vi "arduino-json-messenger.vi"() -> ()   [LabVIEW 2024]
uses:
  <vilib>/Instr/_visa.llb/VISA Configure Serial Port (Instr).vi
panel:
  in  "stop":bool
  in  "Start/Update":bool
  in  "Manual Command Entry":string
  in  "Print Option":string(combo)="all"
  in  "Speed/Offset":i16
  in  "Column":string(combo)="0"
  in  "Row":string(combo)="A"
  in  "Command":T1(ring)
  in  "baud rate 115200":u32=115200
  in  "VISA resource name":refnum<visa-resource-name>="COM29"
  out "Num Bytes Rx":u32
  out "error out":errorcluster
  out "json-cmd":string
  in  "send-cmd":bool
  out "Arduino - Output":string
  in  "exit":bool
  # "ALI-J"
  # "Arduino Labview Interface - JSON"
  # "Data"
  # "{\"cmd\":\"Set offset for fan (at current speed)  -> \"}\n   {\"A0\": -4096 to 4095}\n   {\"C3\": -4096 to 4095}\n\n{\"cmd\":\"Set Global Fan Speed  -> \"}\n   {\"speed\": 0 to 4095}\n\n{\"cmd\":\"Start & Stop Fans  -> \"}\n   {\"start\":0}\n   {\"stop\":0}\n\n{\"cmd\":\"Set Operational Modes ->\"}\n   {\"cal\":\"\"}\n   {\"run\":\"\"}\n\n{\"cmd\":\"View/Save/Delete Data ->\"}\n   {\"save\":\"\"}\n   {\"del\":0 to 4095}\n   {\"print\":\"all\"}\n   {\"print\":\"pwm\"}\n   {\"get\":0 to 4095}\n   {\"help\":\"\"}"
  # "Command Builder"
  # "Serial Options"
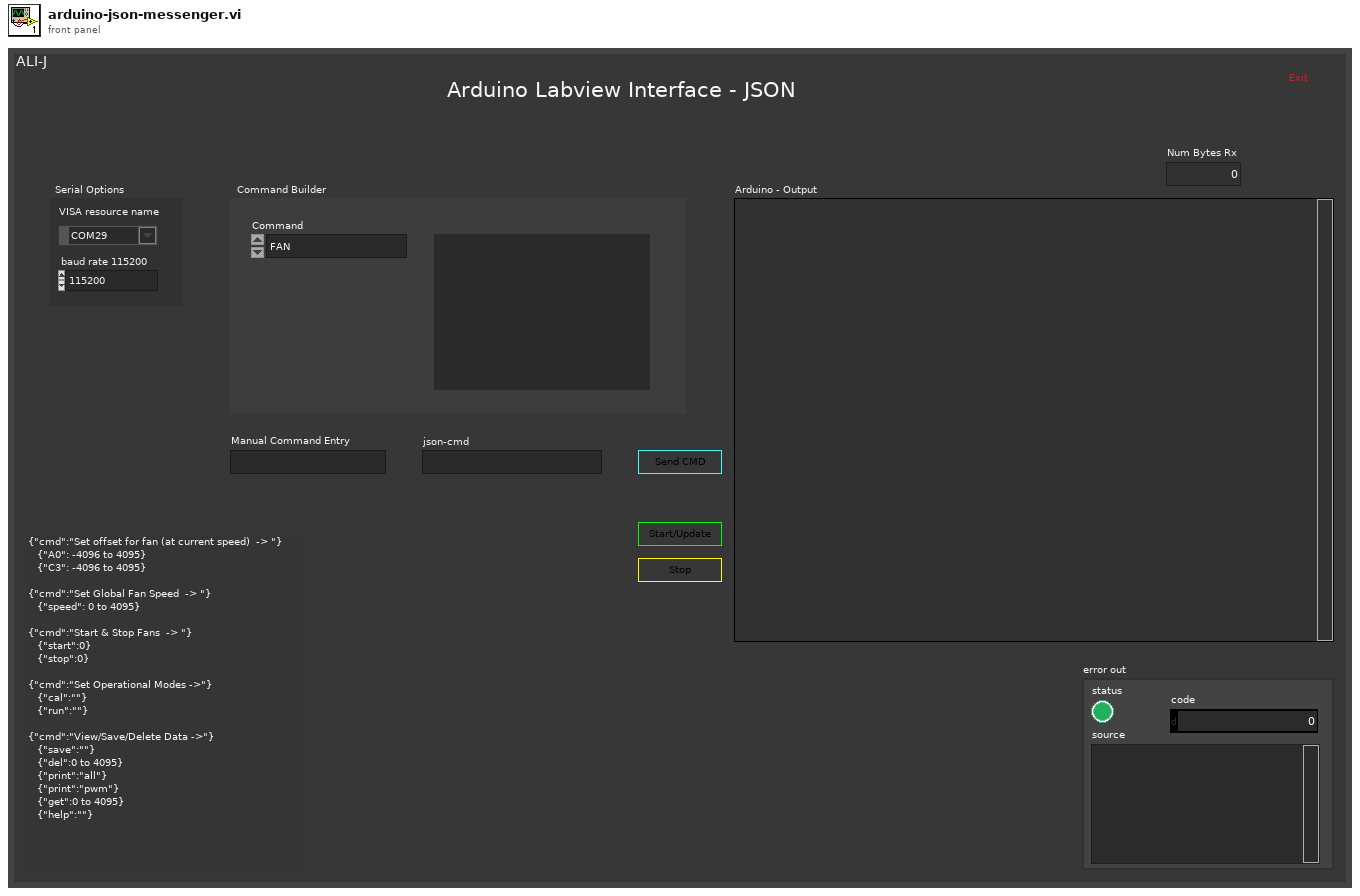
[diagram p1: front panel]
types:
  T1 = enum16{"FAN", "SPEED", "START", "STOP", "CALIBRATE", "RUN", "SAVE", "DELETE", "PRINT", "GET", "HELP", "none"}
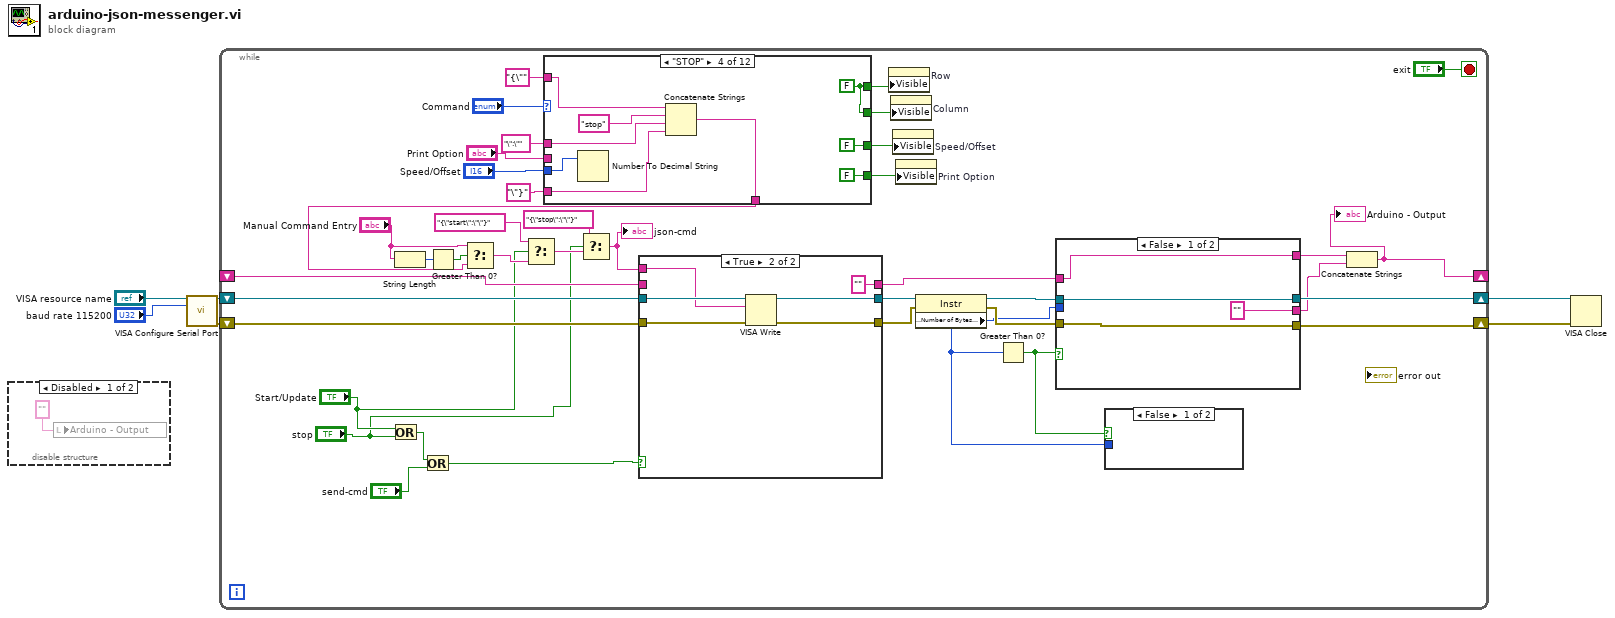
[diagram p0: block diagram]
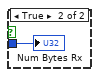
[diagram p3: hidden frame]
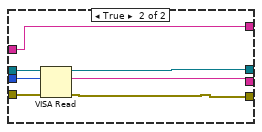
[diagram p4: hidden frame]
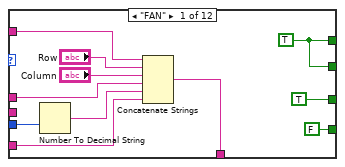
[diagram p6: hidden frame]
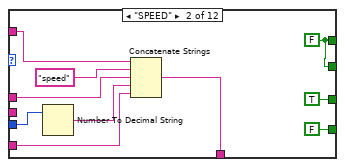
[diagram p7: hidden frame]
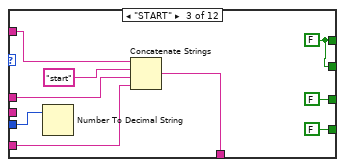
[diagram p8: hidden frame]
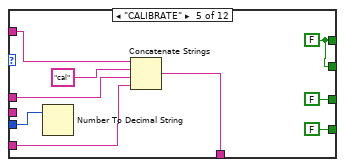
[diagram p9: hidden frame]
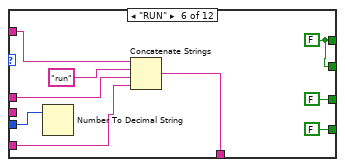
[diagram p10: hidden frame]
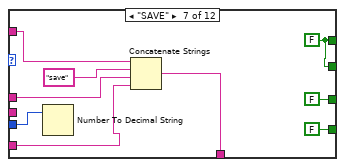
[diagram p11: hidden frame]
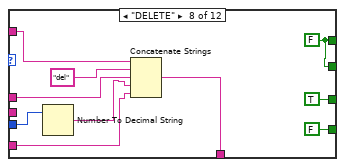
[diagram p12: hidden frame]
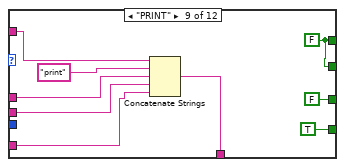
[diagram p13: hidden frame]
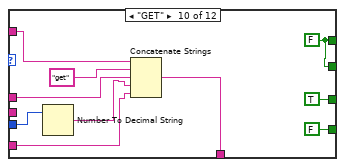
[diagram p14: hidden frame]
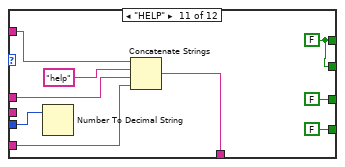
[diagram p15: hidden frame]
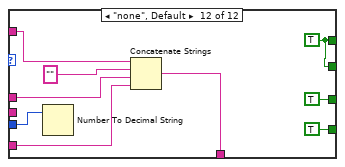
[diagram p16: hidden frame]
diagram:
  n1 = disable-structure shown="Disabled" {
    frame Disabled {
      n2 = local write "Arduino - Output"("" ("string")) -> ()
    }
    frame Enabled {
    }
  }
  n3 = call-poly "VISA Configure Serial Port"("VISA resource name"="VISA resource name", "baud rate (9600)"="baud rate 115200") -> ("VISA resource name out"=w5:refnum<visa-resource-name>, "error out"=w4:errorcluster)  [unwired: 12 in]
  n4 = while {
    shift-right: [w45] -> w3
    shift-left: w5 -> [w37]
    shift-right: [w24] -> w1
    shift-left: w4 -> [w35]
    shift-right: [w25] -> _
    shift-left: _ -> [w26]
    stop <- "exit" stop-if-true
    n5 = Or(x="Start/Update", y="stop") -> (x .or. y?=w16:bool)
    n6 = String Length(string="Manual Command Entry") -> (length=w21:i32)
    n7 = Or(x=w16, y="send-cmd") -> (x .or. y?=w17:bool)
    n8 = Greater Than 0?(x=w21) -> (x > 0?=w20:bool)
    n9 = case shown="\"STOP\"" "Command" {
      tunnel: [w79 w89 w98 w107 w116 w125 w134 w144 w153 w163 w172 w181] -> w42
      tunnel: [w79 w89 w98 w107 w116 w125 w134 w144 w153 w163 w172 w181] -> w41
      tunnel: "Speed/Offset" -> [w75 w85 w94 w103 w112 w121 w130 w140 _ w159 w168 w177]
      tunnel: "{\"" -> [w74 w88 w97 w106 w115 w124 w133 w143 w152 w162 w171 w180]
      tunnel: "\":\"" -> [w73 w86 w95 w104 w113 w122 w131 w141 w150 w160 w169 w178]
      tunnel: [w72 w82 w93 w102 w111 w120 w129 w139 w149 w158 w167 w176] -> w18
      tunnel: "\"}" -> [w71 w83 w92 w101 w110 w119 w128 w136 w147 w155 w165 w175]
      tunnel: [TRUE ("Visible") TRUE ("Visible") FALSE ("Visible") FALSE ("Visible") FALSE ("Visible") FALSE ("Visible") FALSE ("Visible") TRUE ("Visible") FALSE ("Visible") TRUE ("Visible") FALSE ("Visible") TRUE ("Visible")] -> w32
      tunnel: [FALSE ("Visible") FALSE ("Visible") FALSE ("Visible") FALSE ("Visible") FALSE ("Visible") FALSE ("Visible") FALSE ("Visible") FALSE ("Visible") TRUE ("Visible") FALSE ("Visible") FALSE ("Visible") TRUE ("Visible")] -> w23
      tunnel: "Print Option" -> [_ _ _ _ _ _ _ _ w145 _ _ _]
      frame "FAN" {
        w79 = TRUE ("Visible")
        n10 = Number To Decimal String(number=w75) -> (decimal integer string=w76:string)  [unwired: 1 in]
        n11 = Concatenate Strings(w74, "Row", "Column", w73, w76, w71) -> (w72:string)
      }
      frame "SPEED" {
        w89 = FALSE ("Visible")
        n12 = Number To Decimal String(number=w85) -> (decimal integer string=w84:string)  [unwired: 1 in]
        n13 = Concatenate Strings(w88, "speed" ("string"), w86, w84, w83) -> (w82:string)
      }
      frame "START" {
        w98 = FALSE ("Visible")
        n14 = Number To Decimal String(number=w94) -> ()  [unwired: 1 in, 1 out]
        n15 = Concatenate Strings(w97, "start" ("string"), w95, w92) -> (w93:string)
      }
      frame "STOP" {
        w107 = FALSE ("Visible")
        n16 = Number To Decimal String(number=w103) -> ()  [unwired: 1 in, 1 out]
        n17 = Concatenate Strings(w106, "stop" ("string"), w104, w101) -> (w102:string)
      }
      frame "CALIBRATE" {
        w116 = FALSE ("Visible")
        n18 = Number To Decimal String(number=w112) -> ()  [unwired: 1 in, 1 out]
        n19 = Concatenate Strings(w115, "cal" ("string"), w113, w110) -> (w111:string)
      }
      frame "RUN" {
        w125 = FALSE ("Visible")
        n20 = Number To Decimal String(number=w121) -> ()  [unwired: 1 in, 1 out]
        n21 = Concatenate Strings(w124, "run" ("string"), w122, w119) -> (w120:string)
      }
      frame "SAVE" {
        w134 = FALSE ("Visible")
        n22 = Number To Decimal String(number=w130) -> ()  [unwired: 1 in, 1 out]
        n23 = Concatenate Strings(w133, "save" ("string"), w131, w128) -> (w129:string)
      }
      frame "DELETE" {
        w144 = FALSE ("Visible")
        n24 = Number To Decimal String(number=w140) -> (decimal integer string=w137:string)  [unwired: 1 in]
        n25 = Concatenate Strings(w143, "del" ("string"), w141, w137, w136) -> (w139:string)
      }
      frame "PRINT" {
        w153 = FALSE ("Visible")
        n26 = Concatenate Strings(w152, "print" ("string"), w150, w145, w147) -> (w149:string)
      }
      frame "GET" {
        w163 = FALSE ("Visible")
        n27 = Number To Decimal String(number=w159) -> (decimal integer string=w156:string)  [unwired: 1 in]
        n28 = Concatenate Strings(w162, "get" ("string"), w160, w156, w155) -> (w158:string)
      }
      frame "HELP" {
        w172 = FALSE ("Visible")
        n29 = Number To Decimal String(number=w168) -> ()  [unwired: 1 in, 1 out]
        n30 = Concatenate Strings(w171, "help" ("string"), w169, w165) -> (w167:string)
      }
      frame "none", Default {
        w181 = TRUE ("Visible")
        n31 = Number To Decimal String(number=w177) -> ()  [unwired: 1 in, 1 out]
        n32 = Concatenate Strings(w180, "" ("string"), w178, w175) -> (w176:string)
      }
    }
    n33 = Select(t="Manual Command Entry", s=w20, f=w18) -> (s? t:f=w14:string)
    n34 = Select(t="{\"start\":\"\"}", s="Start/Update", f=w14) -> (s? t:f=w13:string)
    n35 = Select(t="{\"stop\":\"\"}", s="stop", f=w13) -> (s? t:f=w12:string)
    "json-cmd" <- w12
    n36 = case shown="True" w17 {
      tunnel: w12 -> [_ w64]
      tunnel: w37 -> [w62 w68]
      tunnel: [w62 w67] -> w36
      tunnel: w35 -> [w61 w66]
      tunnel: [w61 w65] -> w34
      tunnel: [w60 ""] -> w27
      tunnel: w26 -> [w60 _]
      frame False {
      }
      frame True {
        n37 = VISA Write(VISA resource name=w68, write buffer=w64, error in (no error)=w66) -> (VISA resource name out=w67:refnum<visa-resource-name>, error out=w65:errorcluster)  [unwired: 1 out]
      }
    }
    n38 = property on="Row" class="CmbBox"("Visible"=w42) -> ()  [unwired: 2 in, 2 out]
    n39 = property on="Column" class="CmbBox"("Visible"=w41) -> ()  [unwired: 2 in, 2 out]
    n40 = property on="Speed/Offset" class="DigNum (strict)"("Visible"=w32) -> ()  [unwired: 2 in, 2 out]
    n41 = property on="Print Option" class="CmbBox"("Visible"=w23) -> ()  [unwired: 2 in, 2 out]
    n42 = property class="Instr"(reference=w36, error in=w34) -> (reference out=w46:refnum<visa-resource-name>, error out=w47:errorcluster, "Serial Settings:Number of Bytes at Serial Port"=w30:u32)
    n43 = Greater Than 0?(x=w30) -> (x > 0?=w31:bool)
    n44 = case shown="False" w31 {
      tunnel: w47 -> [w51 w59]
      tunnel: w30 -> [_ w58]
      tunnel: w46 -> [w52 w57]
      tunnel: [w52 w56] -> w45
      tunnel: [w51 w55] -> w24
      tunnel: ["" ("read buffer") w54] -> w29
      tunnel: [w49 w53] -> w28
      tunnel: w27 -> [w49 w53]
      frame False {
      }
      frame True {
        n45 = VISA Read(VISA resource name=w57, byte count=w58, error in (no error)=w59) -> (VISA resource name out=w56:refnum<visa-resource-name>, read buffer=w54:string, error out=w55:errorcluster)  [unwired: 1 out]
      }
    }
    n46 = case shown="False" w31 {
      tunnel: w30 -> [_ w48]
      frame False {
      }
      frame True {
        "Num Bytes Rx" <- w48
      }
    }
    n47 = Concatenate Strings(w28, w29) -> (w25:string)
    "Arduino - Output" <- w25
  }
  n48 = VISA Close(VISA resource name=w3, error in (no error)=w1) -> ()  [unwired: 1 out]
